vi "DSF.Transceiver.GE Reflective Memory.Initialize Hardware.vi"(8 "error in (no error)":errorcluster, 11 "DSF GE Reflective Memory Transceiver in":refnum<class "DSF.Transceiver.GE Reflective Memory.lvclass">) -> (0 "error out":errorcluster, 3 "DSF GE Reflective Memory Transceiver out":refnum<class "DSF.Transceiver.GE Reflective Memory.lvclass">)   [LabVIEW 2017, in "DSF.Transceiver.GE Reflective Memory.lvlib" / "DSF.Transceiver.GE Reflective Memory.lvclass"]
uses:
  DSF.Transceiver.GE Reflective Memory.lvclass
  <vilib>/NI/GE Reflective Memory Driver/Typedefs/GE 5565PIORC.Typedef.DMA Wait Mode.ctl
  DSF.Transceiver.GE Reflective Memory.lvclass/DSF.Transceiver.GE Reflective Memory.ctl
  <vilib>/NI/GE Reflective Memory Driver/GE 5565PIORC.lvclass/GE 5565PIORC.ctl
  <vilib>/NI/GE Reflective Memory Driver/Properties/Registers/GE 5565PIORC.Registers.LAS1RR.PCI Address Range.Get.vi
  <vilib>/NI/GE Reflective Memory Driver/Methods/GE 5565PIORC.PXI Interrupts.Enable.vi
  <vilib>/NI/GE Reflective Memory Driver/Properties/Registers/GE 5565PIORC.Registers.DMACSR0.Channel 0 Enable.Set.vi
  <vilib>/NI/GE Reflective Memory Driver/Properties/Registers/GE 5565PIORC.Registers.INTCSR.Local DMA Channel 0 Interrupt Enable.Set.vi
  <vilib>/NI/GE Reflective Memory Driver/Properties/Registers/GE 5565PIORC.Registers.Local Configuration.Read.vi
  <vilib>/NI/GE Reflective Memory Driver/Properties/Registers/GE 5565PIORC.Registers.Local Configuration.Read (U32).vi
  <vilib>/NI/GE Reflective Memory Driver/Properties/Registers/GE 5565PIORC.Registers.Local Configuration.Read (U8).vi
  <vilib>/NI/GE Reflective Memory Driver/Properties/Registers/GE 5565PIORC.Registers.Local Configuration.Write.vi
  <vilib>/NI/GE Reflective Memory Driver/Properties/Registers/GE 5565PIORC.Registers.Local Configuration.Write (U8).vi
  <vilib>/NI/GE Reflective Memory Driver/Methods/GE 5565PIORC.Bit Manipulation.Set Bit.vi
  <vilib>/NI/GE Reflective Memory Driver/Methods/GE 5565PIORC.Bit Manipulation.Set Bit (U8).vi
  <vilib>/NI/GE Reflective Memory Driver/Properties/Registers/GE 5565PIORC.Registers.Local Configuration.Write (U32).vi
  <vilib>/NI/GE Reflective Memory Driver/Methods/GE 5565PIORC.Bit Manipulation.Set Bit (U32).vi
  <vilib>/NI/GE Reflective Memory Driver/Methods/GE 5565PIORC.Registers.Read.vi
  <vilib>/NI/GE Reflective Memory Driver/Methods/GE 5565PIORC.Registers.Read (U32).vi
  <vilib>/NI/GE Reflective Memory Driver/Methods/GE 5565PIORC.Registers.Read (U8).vi
  <vilib>/NI/GE Reflective Memory Driver/Methods/GE 5565PIORC.Registers.Write.vi
  <vilib>/NI/GE Reflective Memory Driver/Methods/GE 5565PIORC.Registers.Write (U8).vi
  <vilib>/NI/GE Reflective Memory Driver/Methods/GE 5565PIORC.Registers.Write (U32).vi
  <vilib>/NI/GE Reflective Memory Driver/GE 5565PIORC.lvclass
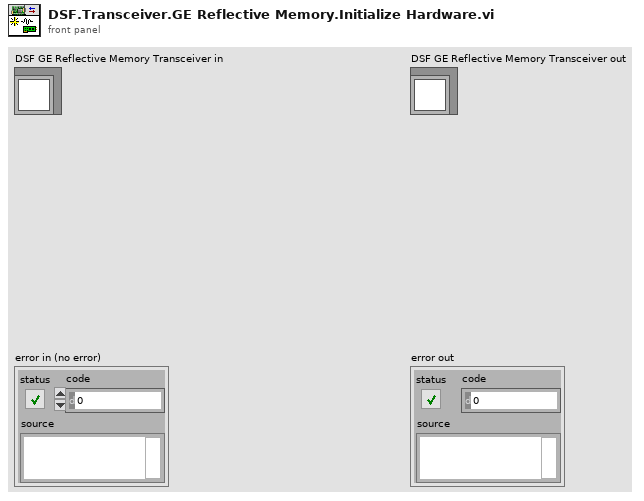
[diagram p1: front panel]
types:
  T1 = typedef "GE 5565PIORC.lvclass/GE 5565PIORC.Typedef.DMA Wait Mode.ctl" = enum16{"Polling", "Interrupt"}
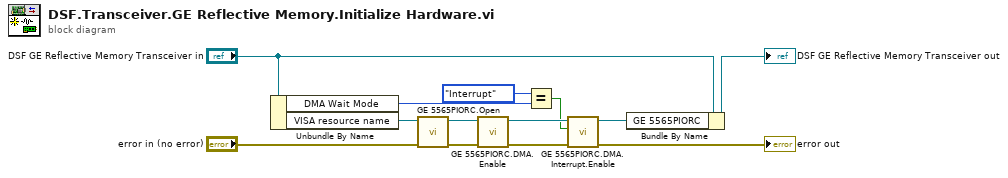
[diagram p0: block diagram]
diagram:
  n1 = Unbundle By Name("DSF GE Reflective Memory Transceiver in") -> ("DMA Wait Mode"=w5:T1, "VISA resource name"=w10:refnum<visa-resource-name>)
  n2 = call <vilib>:"GE 5565PIORC.Open.vi"("error in (no error)"="error in (no error)", "VISA resource name"=w10) -> ("error out"=w9:errorcluster, "GE 5565PIORC"=w8:refnum<class "GE 5565PIORC.lvclass">)  [unwired: 8 in]
  n3 = call <vilib>:"GE 5565PIORC.DMA.Enable.vi"("error in (no error)"=w9, "GE 5565PIORC in"=w8) -> ("error out"=w6:errorcluster, "GE 5565PIORC out"=w7:refnum<class "GE 5565PIORC.lvclass">)  [unwired: 8 in]
  n4 = Equal?(x=GE_5565PIORC.Typedef.DMA_Wait_Mode."Interrupt", y=w5) -> (x = y?=w4:bool)
  n5 = call <vilib>:"GE 5565PIORC.DMA.Interrupt.Enable.vi"("error in (no error)"=w6, "enable (T)"=w4, "GE 5565PIORC in"=w7) -> ("error out"=→"error out":errorcluster, "GE 5565PIORC out"=w1:refnum<class "GE 5565PIORC.lvclass">)  [unwired: 7 in]
  n6 = Bundle By Name(cluster="DSF GE Reflective Memory Transceiver in", "GE 5565PIORC"=w1) -> (→"DSF GE Reflective Memory Transceiver out":refnum<class "DSF.Transceiver.GE Reflective Memory.lvclass">)
